vi "Timestamp.vi"(3 "Anything 3":variant, 4 "Anything 2":variant, 5 "Anything":variant) -> (1 "Start Time":timestamp format="%<%b-%d %H:%M>T")   [LabVIEW 2021]
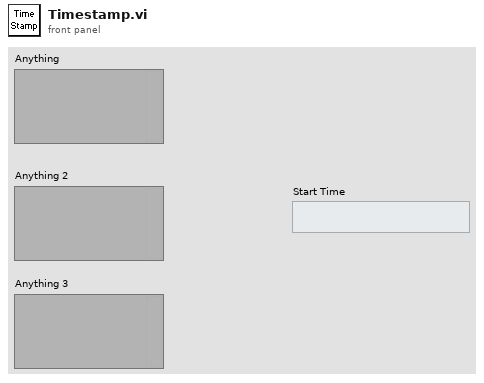
[diagram p1: front panel]
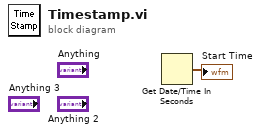
[diagram p0: block diagram]
diagram:
  n1 = Get Date/Time In Seconds() -> (seconds since 1Jan1904=→"Start Time":timestamp)
